vi "UpdateMathsPic.vi"(7 "Path":path=path "not connected", 9 "ref pic in":refnum<vi>, 10 "File Paths":T1={"Local Save Path"=path "C:/Users/cv222/Documents/Jarvis/data", "Newton Save Path"=path "Z:/#Projects/Entanglement/data", "File Name"="test", "LocalSave"=TRUE}, 11 "MathImageCtl":T2) -> (3 "pic out":picture)   [LabVIEW 2019]
uses:
  controls/PltImageControl.ctl
  controls/FilePaths.ctl
  <vilib>/Utility/miscctls.llb/LVPointTypeDef.ctl
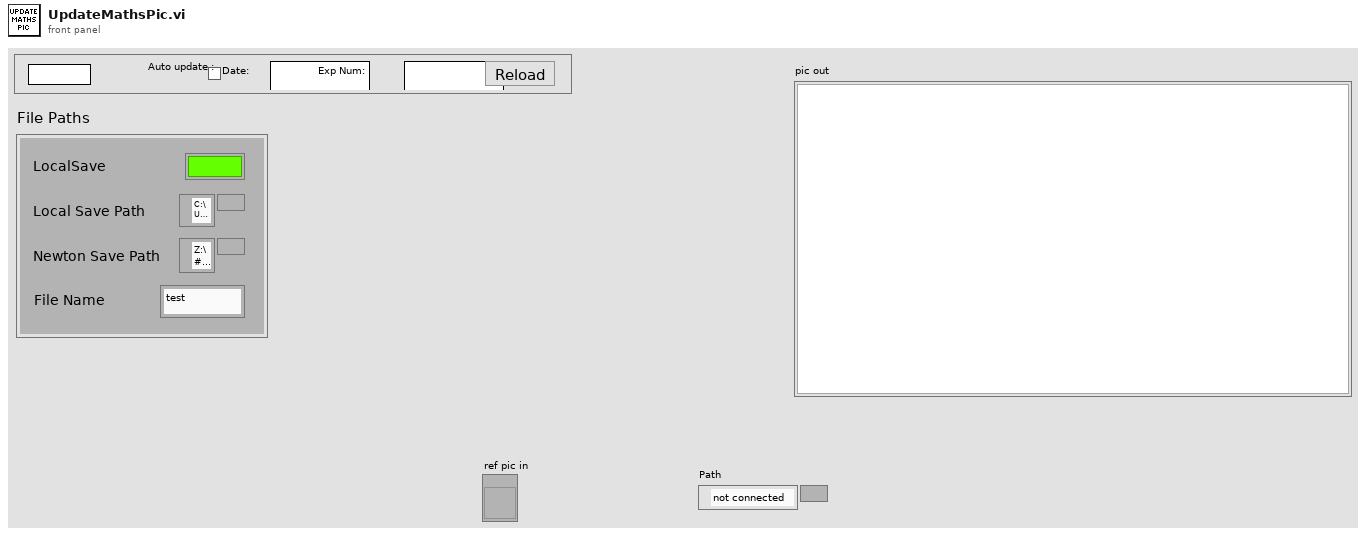
[diagram p1: front panel]
types:
  T1 = typedef "FilePaths.ctl" = cluster{"Local Save Path":path, "Newton Save Path":path, "File Name":string, "LocalSave":bool}
  T2 = typedef "PltImageControl.ctl" = cluster{"Date:":string, "Exp Num:":string, "Reload":bool, "Auto update : ":bool, "String":string}
  T3 = typedef "LVPointTypeDef.ctl" = cluster{"Horizontal":i16, "Vertical":i16}
  T4 = typedef "LVBoundsTypeDef.ctl" = cluster{"Width":u32, "Height":u32}
  T5 = typedef "imagedata.ctl" = cluster{"image type":i32, "image depth":i32, "image":u8[], "mask":u8[], "colors":u32[], "Rectangle":cluster{"left":i16, "top":i16, "right":i16, "bottom":i16}}
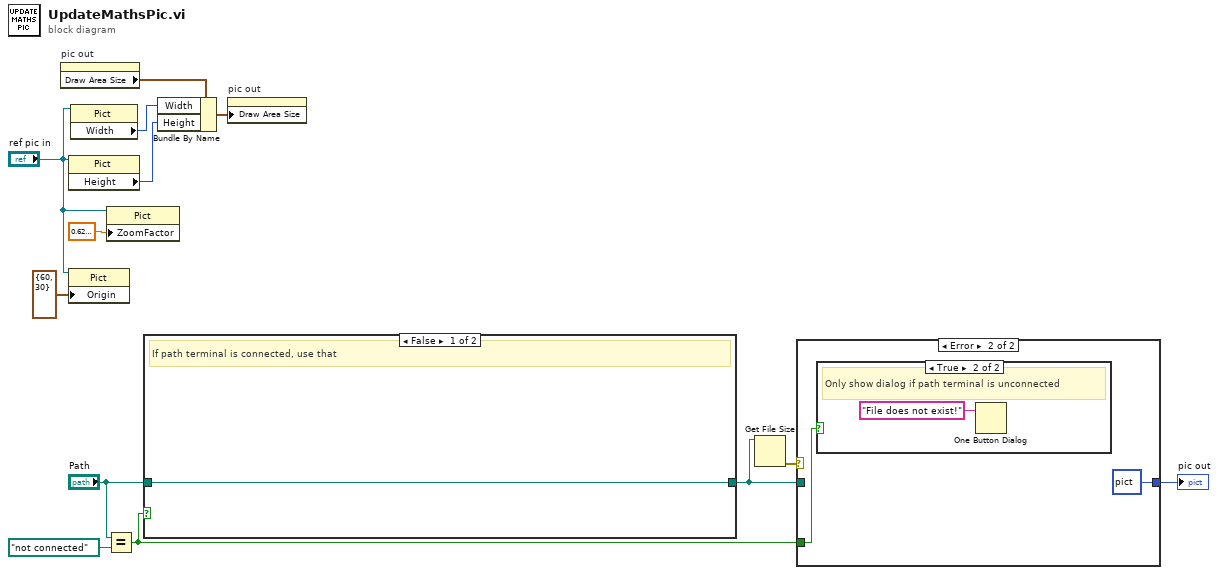
[diagram p0: block diagram]
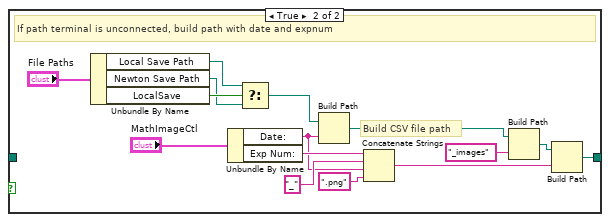
[diagram p2: hidden frame]
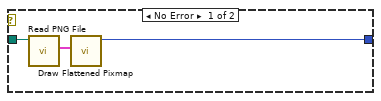
[diagram p3: hidden frame]
diagram:
  n1 = property on="pic out" class="Pict"() -> ("Draw Area Size"=w13:T4)  [unwired: 2 in, 2 out]
  n2 = property class="Pict"(reference="ref pic in") -> ("Height"=w11:u32)  [unwired: 1 in, 2 out]
  n3 = property on="Property Node" class="Pict"(reference="ref pic in", "Origin"=T3 {"Horizontal"=60, "Vertical"=30}) -> ()  [unwired: 1 in, 2 out]
  n4 = property class="Pict"(reference="ref pic in") -> ("Width"=w12:u32)  [unwired: 1 in, 2 out]
  n5 = Equal?(x="Path", y=path "not connected") -> (x = y?=w1:bool)
  n6 = property on="Property Node" class="Pict"(reference="ref pic in", "ZoomFactor"=sgl 0.62 ("Zoom Factor")) -> ()  [unwired: 1 in, 2 out]
  n7 = case shown="False" w1 {
    tunnel: [w14 w23] -> w5
    tunnel: "Path" -> [w14 _]
    frame False {
      # "If path terminal is connected, use that"
    }
    frame True {
      # "Build CSV file path"
      # "If path terminal is unconnected, build path with date and expnum"
      n8 = Unbundle By Name("File Paths") -> ("Local Save Path"=w26:path, "Newton Save Path"=w27:path, "LocalSave"=w28:bool)
      n9 = Unbundle By Name("MathImageCtl") -> ("Date:"=w17:string, "Exp Num:"=w19:string)
      n10 = Select(t=w26, s=w28, f=w27) -> (s? t:f=w29:path)
      n11 = Build Path(base path=w29, name or relative path=w17) -> (appended path=w22:path)
      n12 = Concatenate Strings(w19, "_", w17, ".png" ("string")) -> (w25:string)
      n13 = Build Path(base path=w22, name or relative path="_images") -> (appended path=w20:path)
      n14 = Build Path(base path=w20, name or relative path=w25) -> (appended path=w23:path)
    }
  }
  n15 = Bundle By Name(cluster=w13, "Width"=w12, "Height"=w11) -> (w10:T4)
  n16 = property on="pic out" class="Pict"("Draw Area Size"=w10) -> ()  [unwired: 2 in, 2 out]
  n17 = Get File Size(file=w5) -> (0:w6:errorcluster)  [unwired: 1 in, 2 out]
  n18 = case shown="Error" w6 {
    tunnel: w5 -> [w31 _]
    tunnel: [w30 picture data[5B] ("new picture")] -> w4
    tunnel: w1 -> [_ w33]
    frame No Error {
      n19 = call <vilib>:"Read PNG File.vi"("path to PNG file"=w31) -> ("image data"=w32:T5)  [unwired: 8 in, 2 out]
      n20 = call <vilib>:"Draw Flattened Pixmap.vi"("image data"=w32) -> ("new picture"=w30:picture)  [unwired: 8 in]
    }
    frame Error {
      n21 = case shown="True" w33 {
        frame False {
        }
        frame True {
          # "Only show dialog if path terminal is unconnected"
          n22 = One Button Dialog(message="File does not exist!") -> ()  [unwired: 1 in, 1 out]
        }
      }
    }
  }
  "pic out" <- w4
